vi "proceso6.vi"() -> ()   [LabVIEW 2020]
panel:
  out "proceso 6":T1
  # "pos_inicial_ horizaontal=835\npos_final_horizontal=1105\npos_inicial_ vertical=660\npos_final_vertical=732"
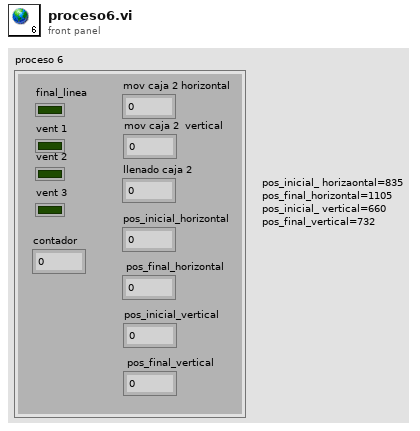
[diagram p1: front panel]
types:
  T1 = cluster{"final_linea":bool, "vent 1":bool, "vent 2":bool, "vent 3":bool, "mov caja 2 horizontal":i32, "llenado caja 2":u8, "pos_inicial_horizontal":dbl, " pos_final_horizontal":dbl, "contador":dbl, "mov caja 2  vertical":i32, "pos_inicial_vertical":dbl, " pos_final_vertical":dbl}
diagram:
